vi "02 Tools, Colors, and Clicks.vi"() -> ()   [LabVIEW 2019]
panel:
  in  "stop":bool
  out "Waveform Chart":dbl(graph)
  in  "Slide":dbl(slide)=5.204081632653061 scale=0.0..10.0
  # "Go to View:Tools Palette to bring it up"
  # "Click on the Axis Labels to edit\nClick on the lowest / highest value of the asix to rescale"
  # "hover over the tools and \nsee what they all do.  Use the\npaint tool to change the color\nof the Chart and Slide"
  # "Right-btn click on the plot and select Properties - and edit..."
  # "Hit Cmd E to see the diagram (code)"
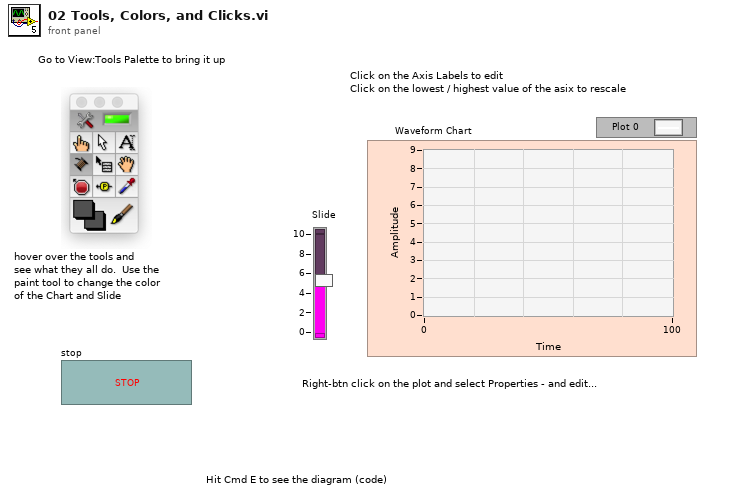
[diagram p1: front panel]
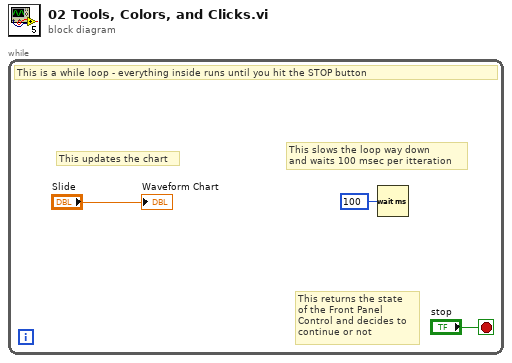
[diagram p0: block diagram]
diagram:
  n1 = while {
    stop <- "stop" stop-if-true
    # "This returns the state\nof the Front Panel \nControl and decides to\ncontinue or not"
    # "This slows the loop way down \nand waits 100 msec per itteration"
    # "This updates the chart"
    # "This is a while loop - everything inside runs until you hit the STOP button"
    n2 = Wait (ms)(milliseconds to wait=u32 100) -> ()  [unwired: 1 out]
    "Waveform Chart" <- "Slide"
  }
